vi "Get Output Channel Values.vi"(11 "Output Process in":refnum<class "Random Process.lvclass">) -> (2 "Output Channel Values":dbl[](array[numeric]), 3 "Output Process out":refnum<class "Random Process.lvclass">)   [LabVIEW 2019, in "TimingDRV Engine.lvlib" / "Random Process.lvclass"]
uses:
  Random Process.lvclass
  Random Process.lvclass/Random Process.ctl
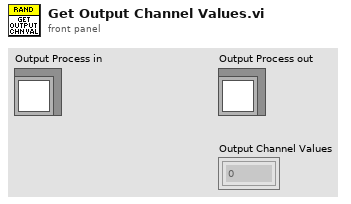
[diagram p1: front panel]
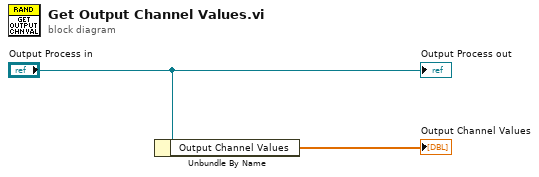
[diagram p0: block diagram]
diagram:
  n1 = Unbundle By Name("Output Process in") -> ("Output Channel Values"=→"Output Channel Values":dbl[])
  "Output Process out" <- "Output Process in"
